vi "testMethod.vi"(8 "error in (no error)":errorcluster, 11 "WasRun in":refnum<class "WasRun.lvclass">) -> (0 "error out":errorcluster, 3 "WasRun out":refnum<class "WasRun.lvclass">)   [LabVIEW 2013, in "WasRun.lvclass"]
uses:
  WasRun.lvclass
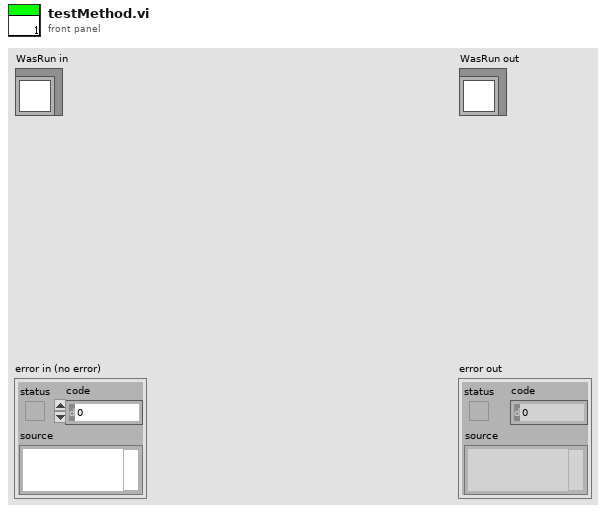
[diagram p1: front panel]
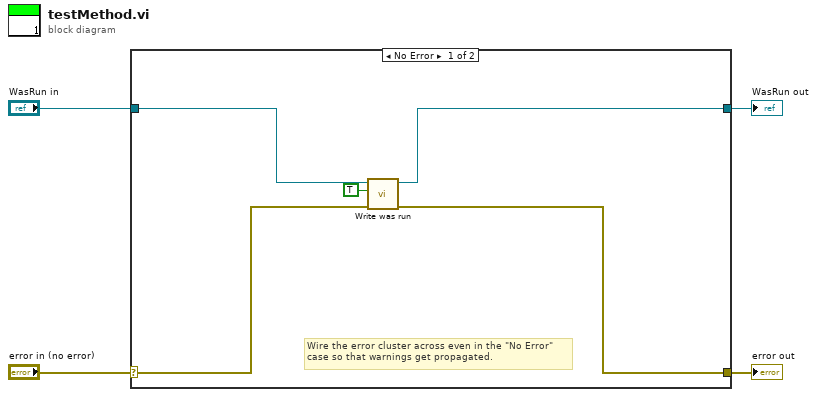
[diagram p0: block diagram]
diagram:
  n1 = case shown="No Error" "error in (no error)" {
    selector: "error in (no error)" -> [w6 w11]
    tunnel: [w5 w11] -> w3
    tunnel: [w7 w10] -> w1
    tunnel: "WasRun in" -> [w8 w10]
    frame No Error {
      # "Wire the error cluster across even in the \"No Error\"\ncase so that warnings get propagated."
      n2 = call-dynamic "Write was run.vi"("error in (no error)"=w6, "was run"=TRUE, "WasRun in"=w8) -> ("error out"=w5:errorcluster, "WasRun out"=w7:refnum<class "WasRun.lvclass">)  [unwired: 7 in]
    }
    frame Error {
    }
  }
  "error out" <- w3
  "WasRun out" <- w1
